vi "InsertOneRecordTo2DListCtrl.vi"(10 "배열":string[](array[string]), 11 "testcaselist in":refnum<vi>) -> (3 "testcaselist out":refnum<vi>)   [LabVIEW 2018, in "Library-Ctrl.lvlib"]
uses:
  Library-Ctrl.lvlib
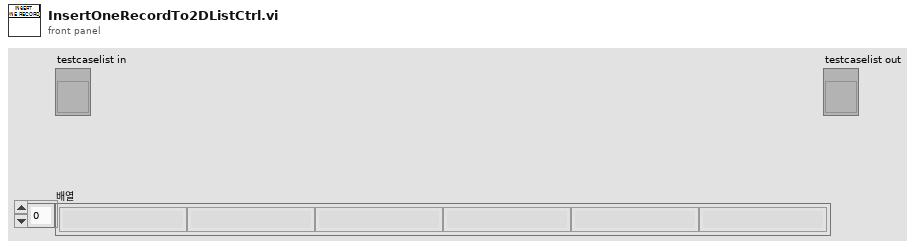
[diagram p1: front panel]
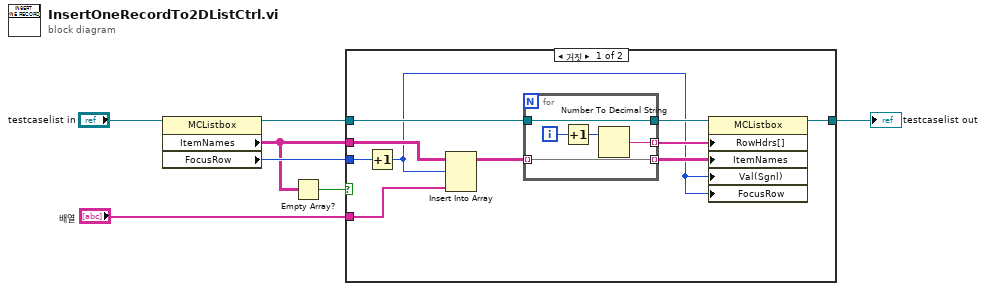
[diagram p0: block diagram]
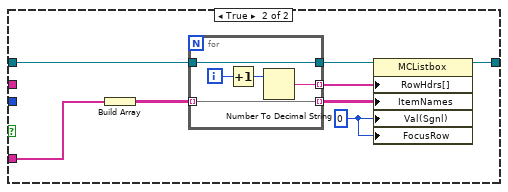
[diagram p2: hidden frame]
diagram:
  n1 = property class="MCListbox"(reference="testcaselist in") -> (reference out=w5:refnum<vi>, "ItemNames"=w3:string[][], "FocusRow"=w4:i32)  [unwired: 1 in, 1 out]
  n2 = Empty Array?(array=w3) -> (empty?=w6:bool)
  n3 = case shown="거짓" w6 {
    tunnel: w5 -> [w12 w29]
    tunnel: w4 -> [w9 _]
    tunnel: w3 -> [w17 _]
    tunnel: "배열" -> [w16 w30]
    tunnel: [w10 w24] -> w1
    frame False {
      n4 = Increment(x=w9) -> (x+1=w8:i32)
      n5 = Insert Into Array(array=w17, index (row)=w8, new element=w16) -> (w11:string[][])  [unwired: 1 in]
      n6 = for {
        tunnel: w12 -> [w22]
        tunnel: [w22] -> w15
        tunnel: [w19] -> w14 mode=indexing
        tunnel: [w18] -> w13 mode=indexing
        tunnel: w11 -> [w18] mode=indexing
        i -> [w21]
        n7 = Increment(x=w21) -> (x+1=w20:i32)
        n8 = Number To Decimal String(number=w20) -> (decimal integer string=w19:string)  [unwired: 1 in]
      }
      n9 = property class="MCListbox"(reference=w15, "RowHdrs[]"=w14, "ItemNames"=w13, "Val(Sgnl)"=w8, "FocusRow"=w8) -> (reference out=w10:refnum<vi>)  [unwired: 1 in, 1 out]
    }
    frame True {
      w23 = u16 0
      n10 = Build Array(w30) -> (w25:string[][])
      n11 = for {
        tunnel: w29 -> [w35]
        tunnel: [w35] -> w28
        tunnel: [w32] -> w27 mode=indexing
        tunnel: [w31] -> w26 mode=indexing
        tunnel: w25 -> [w31] mode=indexing
        i -> [w34]
        n12 = Increment(x=w34) -> (x+1=w33:i32)
        n13 = Number To Decimal String(number=w33) -> (decimal integer string=w32:string)  [unwired: 1 in]
      }
      n14 = property class="MCListbox"(reference=w28, "RowHdrs[]"=w27, "ItemNames"=w26, "Val(Sgnl)"=w23, "FocusRow"=w23) -> (reference out=w24:refnum<vi>)  [unwired: 1 in, 1 out]
    }
  }
  "testcaselist out" <- w1
